vi "Configure Digits for Display.vi"(8 "error in (no error)":errorcluster, 9 "Display Digits (5)":u32=5, 10 "Function (0: Volts)":u16(ring) items=["Volts", "Current", "Resistance", "Digitize Voltage", "Digitize Current"], 11 "VISA resource name":refnum<visa-resource-name>) -> (0 "error out":errorcluster, 3 "VISA resource name out":refnum<visa-resource-name>)   [LabVIEW 2021, in "Keithley 2450.lvlib"]
doc: "Determines the number of digits that are displayed for measurements.\n\n<B>The Digitize Voltage and Digitize Current functions are only valid on the 2461</B>"
uses:
  <instrlib>/Keithley 2450/Keithley 2450.lvlib
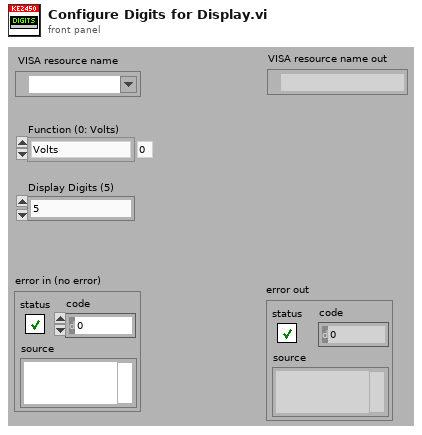
[diagram p1: front panel]
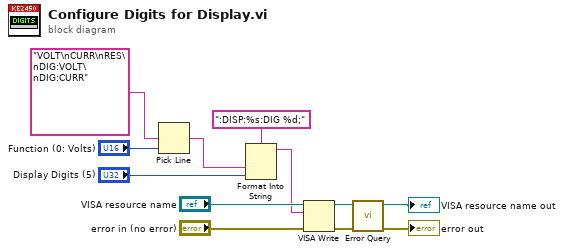
[diagram p0: block diagram]
diagram:
  n1 = Pick Line(multi-line string="VOLT\nCURR\nRES\nDIG:VOLT\nDIG:CURR", line index="Function (0: Volts)") -> (output string=w1:string)  [unwired: 1 in]
  n2 = Format Into String(format string=":DISP:%s:DIG %d;", w1, "Display Digits (5)") -> (resulting string=w5:string)  [unwired: 2 in, 1 out]
  n3 = VISA Write(VISA resource name="VISA resource name", write buffer=w5, error in (no error)="error in (no error)") -> (VISA resource name out=w10:refnum<visa-resource-name>, error out=w7:errorcluster)  [unwired: 1 out]
  n4 = call <instrlib>:"Error Query.vi"("error in (no error)"=w7, "VISA resource name"=w10) -> ("error out"=→"error out":errorcluster, "VISA resource name out"=→"VISA resource name out":refnum<visa-resource-name>)  [unwired: 8 out]
